vi "Smooth Background CDBL.vi"(8 "Error In":errorcluster, 9 "HP F":dbl format="%#_6p", 10 "LP  F":dbl=0.001 format="%#_6p", 11 "Data":cdb[](array[numeric])) -> (0 "Error Out":errorcluster, 3 "Data out":cdb[](array[numeric]))   [LabVIEW 2016]
uses:
  <vilib>/Analysis/3filter.llb/Filter Structure Type.ctl
  <vilib>/measure/macond.llb/IIR Filter for 1 Chan (CDB).vi
  <vilib>/measure/NI_MAPro.lvlib
  <vilib>/Analysis/NI_AALBase.lvlib
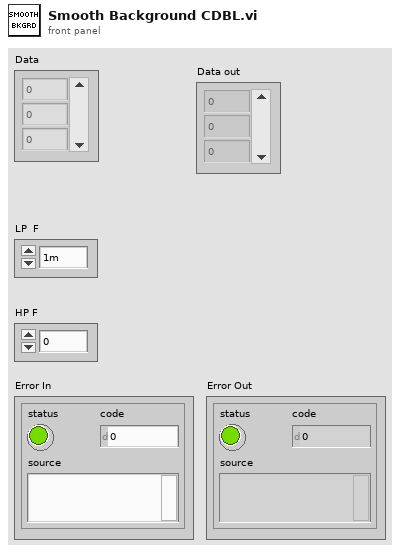
[diagram p1: front panel]
types:
  T1 = typedef "NI_AALBase.lvlib/Filter Structure Type.ctl" = u16
  T2 = cluster{"Topology":enum16{"Off", "Butterworth", "Chebyshev", "Inverse Chebyshev", "Elliptic", "Bessel"}, "Type":enum16{"Lowpass", "Highpass", "Bandpass", "Bandstop"}, "Order":i32, "Lower Fc":dbl, "Upper Fc":dbl, "PB Ripple":dbl, "SB Attenuation":dbl}
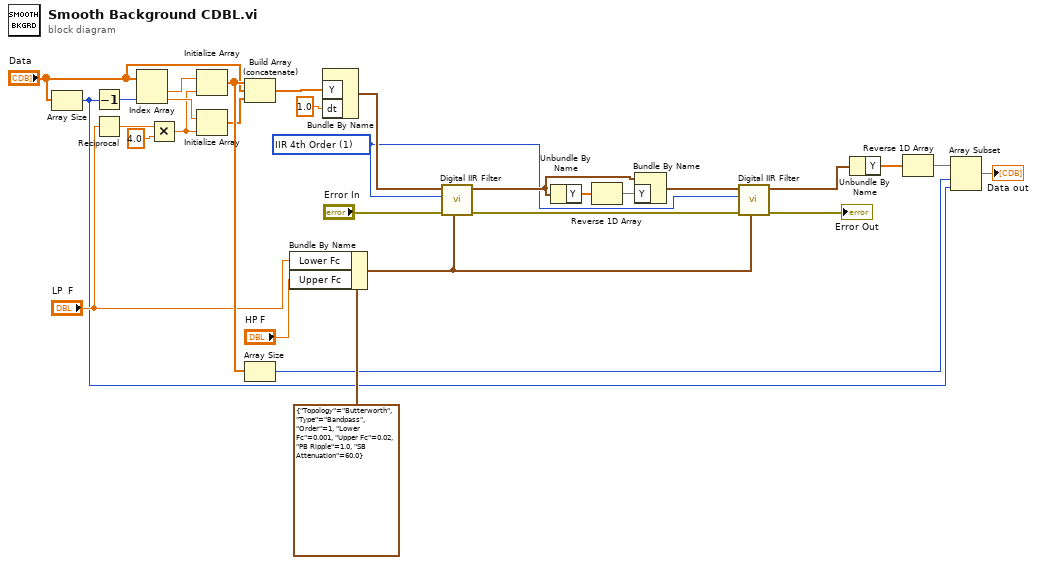
[diagram p0: block diagram]
diagram:
  w15 = T1 1 items=["IIR 2nd Order"=0, "IIR 4th Order"=1, "Auto Select"=10] ("filter structure option")
  n1 = Array Size(array="Data") -> (size(s)=w7:i32)
  n2 = Decrement(x=w7) -> (x-1=w6:i32)
  n3 = Reciprocal(x="LP  F") -> (1/x=w26:dbl)
  n4 = Index Array(array="Data", index #2=w6) -> (element #1=w28:cdb, element #2=w5:cdb)  [unwired: 1 in]
  n5 = Multiply(x=w26, y=4.0) -> (x*y=w4:dbl)
  n6 = Initialize Array(w28, w4) -> (w30:cdb[])
  n7 = Initialize Array(w5, w4) -> (w3:cdb[])
  n8 = Build Array (concatenate)(w30, "Data", w3) -> (w29:cdb[])
  n9 = Array Size(array=w30) -> (size(s)=w10:i32)
  n10 = Bundle By Name(cluster=T2 {"Topology"=enum."Butterworth", "Type"=enum."Bandpass", "Order"=1, "Lower Fc"=0.001, "Upper Fc"=0.02, "PB Ripple"=1.0, "SB Attenuation"=60.0} ("IIR filter specifications"), "Lower Fc"="LP  F", "Upper Fc"="HP F") -> (w16:T2)
  n11 = Bundle By Name("Y"=w29, "dt"=1.0) -> (w24:waveform(cdb))  [unwired: 1 in]
  n12 = call-poly <vilib>:"Digital IIR Filter.vi"("IIR filter specifications"=w16, "error in (no error)"="Error In", "filter structure option"=w15, "signal in"=w24) -> ("error out"=w14:errorcluster, "signal out"=w19:waveform(cdb))  [unwired: 5 in, 1 out]
  n13 = Unbundle By Name(w19) -> ("Y"=w20:cdb[])
  n14 = Reverse 1D Array(array=w20) -> (reversed array=w18:cdb[])
  n15 = Bundle By Name(cluster=w19, "Y"=w18) -> (w17:waveform(cdb))
  n16 = call-poly <vilib>:"Digital IIR Filter.vi"("IIR filter specifications"=w16, "error in (no error)"=w14, "filter structure option"=w15, "signal in"=w17) -> ("error out"=→"Error Out":errorcluster, "signal out"=w12:waveform(cdb))  [unwired: 5 in, 1 out]
  n17 = Unbundle By Name(w12) -> ("Y"=w13:cdb[])
  n18 = Reverse 1D Array(array=w13) -> (reversed array=w11:cdb[])
  n19 = Array Subset(array=w11, index=w10, length=w7) -> (→"Data out":cdb[])
